vi "BuildConfigWord.vi"(11 "NewVal":T1) -> (3 "string":string)   [LabVIEW 2020, in "CTI-Peripheral.lvlib" / "Grove An In ADS1115.lvclass"]
uses:
  Grove An In ADS1115.lvclass
  ConfigData.ctl
  ADS1115Mode.ctl
  ADS1115Mux.ctl
  ADS1115DataRate.ctl
  ADS1115PGA.ctl
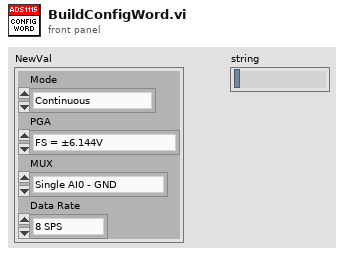
[diagram p1: front panel]
types:
  T1 = typedef "CTI-Peripheral.lvlib/Grove An In ADS1115.lvclass/ConfigData.ctl" = cluster{"Mode":T2, "MUX":T3, "Data Rate":T4, "PGA":T5}
  T2 = typedef "CTI-Peripheral.lvlib/Grove An In ADS1115.lvclass/ADS1115Mode.ctl" = enum16{"Continuous", "Single-Shot"}
  T3 = typedef "CTI-Peripheral.lvlib/Grove An In ADS1115.lvclass/ADS1115Mux.ctl" = enum16{"Single AI0 - GND", "Single AI1 - GND", "Single AI2 - GND", "Single AI3 - GND"}
  T4 = typedef "CTI-Peripheral.lvlib/Grove An In ADS1115.lvclass/ADS1115DataRate.ctl" = enum16{"8 SPS", "16 SPS", "32 SPS", "64 SPS", "128 SPS", "250 SPS", "475 SPS", "860 SPS"}
  T5 = typedef "CTI-Peripheral.lvlib/Grove An In ADS1115.lvclass/ADS1115PGA.ctl" = enum16{"FS = ±6.144V", "FS = ±4.096V", "FS = ±2.048V", "FS = ±1.024V", "FS = ±0.512V", "FS = ±0.256V"}
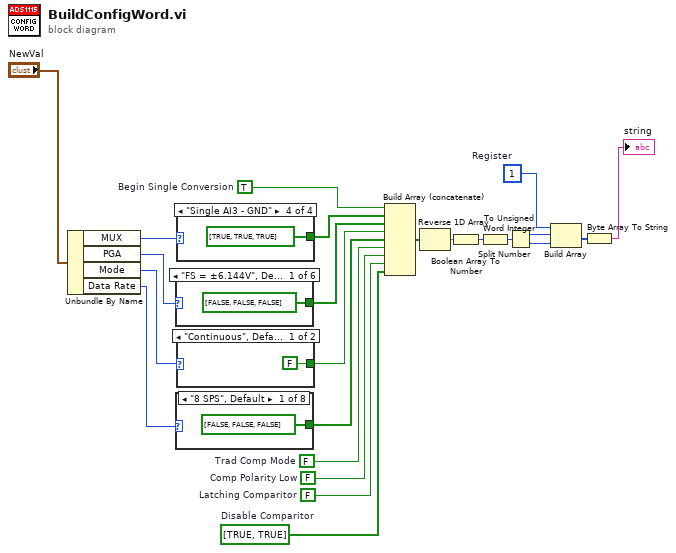
[diagram p0: block diagram]
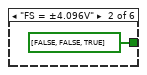
[diagram p2: hidden frame]
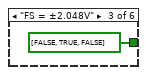
[diagram p3: hidden frame]
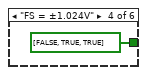
[diagram p4: hidden frame]
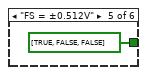
[diagram p5: hidden frame]
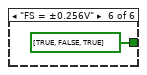
[diagram p6: hidden frame]
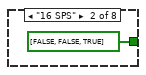
[diagram p7: hidden frame]
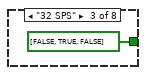
[diagram p8: hidden frame]
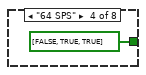
[diagram p9: hidden frame]
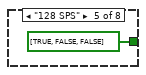
[diagram p10: hidden frame]
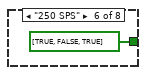
[diagram p11: hidden frame]
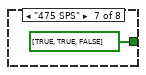
[diagram p12: hidden frame]
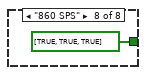
[diagram p13: hidden frame]
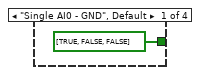
[diagram p14: hidden frame]
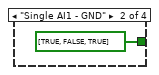
[diagram p15: hidden frame]
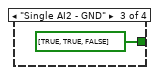
[diagram p16: hidden frame]
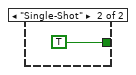
[diagram p17: hidden frame]
diagram:
  w1 = u8 1  # Register
  w15 = bool[] [TRUE, TRUE]  # Disable Comparitor
  w14 = FALSE  # Latching Comparitor
  w13 = FALSE  # Comp Polarity Low
  w12 = FALSE  # Trad Comp Mode
  w5 = TRUE  # Begin Single Conversion
  n1 = Unbundle By Name("NewVal") -> ("MUX"=w3:T3, "PGA"=w4:T5, "Mode"=w8:T2, "Data Rate"=w10:T4)
  n2 = case shown="\"FS = ±6.144V\", Default" w4 {
    tunnel: [bool[] [FALSE, FALSE, FALSE] bool[] [FALSE, FALSE, TRUE] bool[] [FALSE, TRUE, FALSE] bool[] [FALSE, TRUE, TRUE] bool[] [TRUE, FALSE, FALSE] bool[] [TRUE, FALSE, TRUE]] -> w7
    frame "FS = ±6.144V", Default {
    }
    frame "FS = ±4.096V" {
    }
    frame "FS = ±2.048V" {
    }
    frame "FS = ±1.024V" {
    }
    frame "FS = ±0.512V" {
    }
    frame "FS = ±0.256V" {
    }
  }
  n3 = case shown="\"8 SPS\", Default" w10 {
    tunnel: [bool[] [FALSE, FALSE, FALSE] bool[] [FALSE, FALSE, TRUE] bool[] [FALSE, TRUE, FALSE] bool[] [FALSE, TRUE, TRUE] bool[] [TRUE, FALSE, FALSE] bool[] [TRUE, FALSE, TRUE] bool[] [TRUE, TRUE, FALSE] bool[] [TRUE, TRUE, TRUE]] -> w11
    frame "8 SPS", Default {
    }
    frame "16 SPS" {
    }
    frame "32 SPS" {
    }
    frame "64 SPS" {
    }
    frame "128 SPS" {
    }
    frame "250 SPS" {
    }
    frame "475 SPS" {
    }
    frame "860 SPS" {
    }
  }
  n4 = case shown="\"Single AI3 - GND\"" w3 {
    tunnel: [bool[] [TRUE, FALSE, FALSE] bool[] [TRUE, FALSE, TRUE] bool[] [TRUE, TRUE, FALSE] bool[] [TRUE, TRUE, TRUE]] -> w6
    frame "Single AI0 - GND", Default {
    }
    frame "Single AI1 - GND" {
    }
    frame "Single AI2 - GND" {
    }
    frame "Single AI3 - GND" {
    }
  }
  n5 = case shown="\"Continuous\", Default" w8 {
    tunnel: [FALSE TRUE] -> w9
    frame "Continuous", Default {
    }
    frame "Single-Shot" {
    }
  }
  n6 = Build Array (concatenate)(w5, w6, w7, w9, w11, w12, w13, w14, w15) -> (w16:bool[])
  n7 = Reverse 1D Array(array=w16) -> (reversed array=w21:bool[])
  n8 = Boolean Array To Number(Boolean array=w21) -> (number=w17:u32)
  n9 = To Unsigned Word Integer(number=w17) -> (unsigned 16bit integer=w18:u16)
  n10 = Split Number(x=w18) -> (hi(x)=w22:u8, lo(x)=w23:u8)
  n11 = Build Array(w1, w22, w23) -> (w19:u8[])
  n12 = Byte Array To String(unsigned byte array=w19) -> (string=→"string":string)
